vi "status of relay.vi"() -> ()   [LabVIEW 2020]
panel:
  in  "status of relay":bool
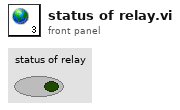
[diagram p1: front panel]
diagram:
